vi "LWXPS_MoveSlice.vi"(0 "XPS Reference IN":refnum<k24>, 5 "Y target position in µm":dbl, 7 "X target position in µm":dbl, 9 "Scan-angle in µrad":dbl, 11 "LabVIEW error IN":errorcluster) -> (4 "XPS Reference OUT":refnum<k24>, 6 "Returned error code":i32, 8 "XPS Error String":string, 15 "LabVIEW error OUT":errorcluster)   [LabVIEW 2014]
uses:
  D:/XPSQ8_LabView_Library/Development/Source/Dll/Newport.XPS.CommandInterface.dll
  Dll/Newport.XPS.CommandInterface.dll
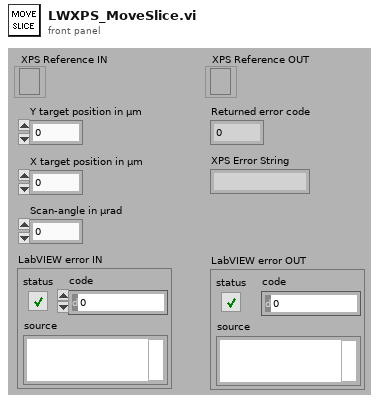
[diagram p1: front panel]
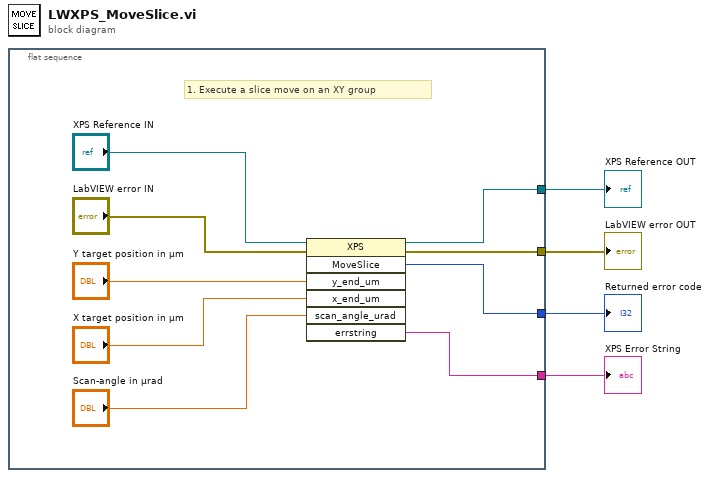
[diagram p0: block diagram]
diagram:
  n1 = flat-sequence {
    tunnel: [w11] -> w4
    tunnel: [w13] -> w3
    tunnel: [w10] -> w2
    tunnel: [w6] -> w1
    frame #0 {
      # "1. Execute a slice move on an XY group"
      n2 = invoke class="XPS" method="MoveSlice"(reference="XPS Reference IN", error in="LabVIEW error IN", "y_end_um"="Y target position in µm", "x_end_um"="X target position in µm", "scan_angle_urad"="Scan-angle in µrad") -> (reference out=w11:refnum<k24>, error out=w13:errorcluster, "MoveSlice"=w10:i32, "errstring"=w6:string)  [unwired: 2 in, 3 out]
    }
  }
  "XPS Reference OUT" <- w4
  "LabVIEW error OUT" <- w3
  "Returned error code" <- w2
  "XPS Error String" <- w1
